vi "Test.vi"   [LabVIEW 2020]
uses:
  Libraries/Acquisition/SignalConfig--cluster.ctl
  Libraries/DataBase/DataBase.lvlib
types:
  T1 = typedef "SignalConfig--cluster.ctl" = cluster{"VPP":i32, "Frecuency":dbl, "Offset":dbl, "signal type":enum16{"Sine Wave", "Triangle Wave", "Square Wave", "Sawtooth Wave"}}
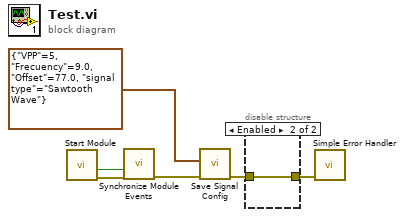
[diagram p0: block diagram]
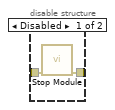
[diagram p2: hidden frame]
diagram:
  n1 = call "Start Module.vi"() -> ("error out"=w6:errorcluster, "Wait for Event Sync?"=w5:bool)  [unwired: 8 in, 2 out]
  n2 = call "Synchronize Module Events.vi"("error in (no error)"=w6, "Wait for Event Sync?"=w5) -> ("error out"=w4:errorcluster)  [unwired: 9 in]
  n3 = call "Save Signal Config.vi"("error in"=w4, "SignalConfig"=T1 {"VPP"=5, "Frecuency"=9.0, "Offset"=77.0, "signal type"=enum."Sawtooth Wave"}) -> ("error out"=w3:errorcluster)  [unwired: 9 in]
  n4 = disable-structure shown="Enabled" {
    disable-tunnel: w3 -> [w8 w9]
    disable-tunnel: [w7 w9] -> w1
    frame Disabled {
      n5 = call "Stop Module.vi"("error in (no error)"=w8) -> ("error out"=w7:errorcluster)  [unwired: 10 in]
    }
    frame Enabled {
    }
  }
  n6 = call <vilib>:"Simple Error Handler.vi"("error in (no error)"=w1) -> ()  [unwired: 4 in, 5 out]
